vi "Stop and Wait on Loop.vi"(8 "error in (no error)":errorcluster, 11 "WebProjectWatcher in":refnum<class "WebProjectWatcher.lvclass">) -> (0 "error out":errorcluster, 3 "WebProjectWatcher out":refnum<class "WebProjectWatcher.lvclass">)   [LabVIEW 2020, in "PicoG-Processor.lvlib" / "WebProjectWatcher.lvclass"]
uses:
  WebProjectWatcher.lvclass
  WebProjectWatcher.lvclass/WebProjectWatcher.ctl
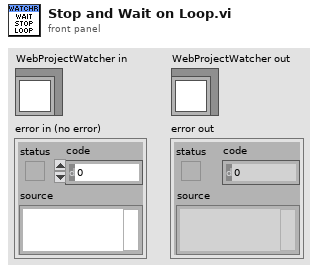
[diagram p1: front panel]
types:
  T1 = typedef "PicoG-Processor.lvlib/WebProjectWatcher.lvclass/Ref Data.ctl" = cluster{"Builds Callbacks":T2[], "Project Path":path, "Close":bool}
  T2 = typedef "PicoG-Processor.lvlib/WebProjectWatcher.lvclass/Builds Callback.ctl" = cluster{"Callback":refnum<vi>, "Owner":refnum<class>}
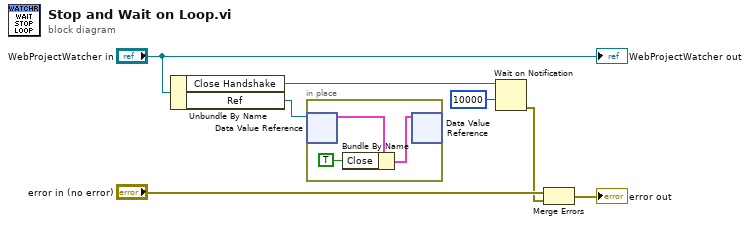
[diagram p0: block diagram]
diagram:
  n1 = Unbundle By Name("WebProjectWatcher in") -> ("Close Handshake"=w4:refnum<notifier>, "Ref"=w6:refnum<data-value>)
  n2 = in-place {
    n3 = in-place-dvr #1(w6) -> (w10:T1)  [unwired: 1 out]
    n4 = Bundle By Name(cluster=w10, "Close"=TRUE) -> (w9:T1)
    n5 = in-place-dvr #1(w9) -> ()  [unwired: 2 out]
  }
  n6 = Wait on Notification(notifier=w4, timeout in ms (-1)=10000) -> (error out=w1:errorcluster)  [unwired: 2 in, 3 out]
  n7 = Merge Errors("error in (no error)", w1) -> (→"error out":errorcluster)
  "WebProjectWatcher out" <- "WebProjectWatcher in"
